vi "DIO64 Out Write.vi"(0 "board in":u16 format="%.0x", 5 "data":u16[][](array[numeric]) format="%.0x", 7 "Out Status":T1 {"startTime0" format="%.0x"; "startTime1" format="%.0x"; "cur trans" format="%.0x"; "cur reps" format="%.0x"; "#trans" format="%.0x"; "reps" format="%.0x"; "stopTime1" format="%.0x"; "stopTime0" format="%.0x"; "pktsize" format="%.0x"; "flags" format="%.0x"; "AICurrent" format="%.0x"; "startControl" format="%.0x"; "stopControl" format="%.0x"; "AIControl" format="%.0x"; "clkControl" format="%.0x"; "time0" format="%.0x"; "time1" format="%.0x"; "ticks" format="%.0x"; "readPtr" format="%.0x"; "writePtr" format="%.0x"; "fifo0" format="%.0x"; "fifoSize" format="%.0x"; "portCount" format="%.0x"}, 11 "error in (no error)":errorcluster) -> (4 "board out":u16 format="%.0x", 15 "error out":errorcluster)   [LabVIEW 2012]
doc: "DIO64 Out Write fills the output buffer with the data specified.\n\nCopyright (c) 2002 Viewpoint Systems Inc. All Rights Reserved"
uses:
  DIO64 Out Status.ctl
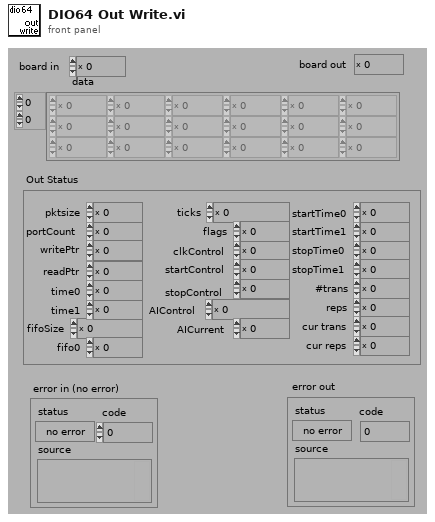
[diagram p1: front panel]
types:
  T1 = typedef "DIO64 Out Status.ctl" = cluster{"pktsize":u16, "portCount":u16, "writePtr":u16, "readPtr":u16, "time0":u16, "time1":u16, "fifoSize":u32, "fifo0":u16, "ticks":u32, "flags":u16, "clkControl":u16, "startControl":u16, "stopControl":u16, "AIControl":u32, "AICurrent":u16, "startTime0":u16, "startTime1":u16, "stopTime0":u16, "stopTime1":u16, "#trans":u16, "reps":u16, "cur trans":u16, "cur reps":u16}
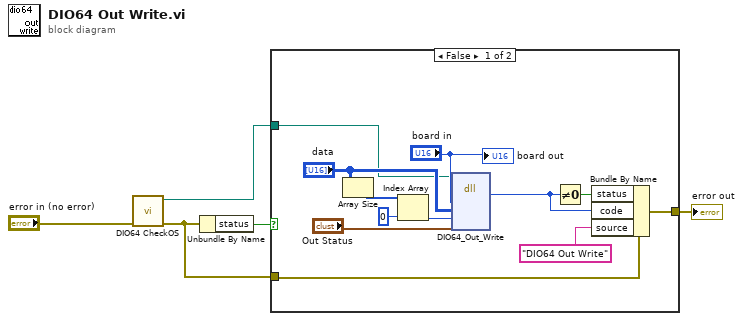
[diagram p0: block diagram]
diagram:
  n1 = call "DIO64 CheckOS.vi"("error in"="error in (no error)") -> ("error out"=w2:errorcluster, "path in"=w1:path)  [unwired: 9 in]
  n2 = Unbundle By Name(w2) -> ("status"=w5:bool)
  n3 = case shown="False" w5 {
    tunnel: w2 -> [w17 w18]
    tunnel: [w14 w18] -> w4
    tunnel: w1 -> [w6 _]
    frame False {
      n4 = Array Size(array="data") -> (size(s)=w9:i32[])
      n5 = Index Array(array=w9, index=0) -> (element=w10:i32)
      n6 = dll-call lib="C:/DIO64Visa/DLL/DIO64_Visa32/Debug/DIO64_Visa32.dll" fn="DIO64_Out_Write"(path in=w6, "board"="board in", "buffer"="data", "bufferSize"=w10, "status"="Out Status") -> ("return type"=w15:i32)  [unwired: 6 in, 2 out]
      n7 = Not Equal To 0?(x=w15) -> (x != 0?=w16:bool)
      n8 = Bundle By Name(cluster=w17, "status"=w16, "code"=w15, "source"="DIO64 Out Write") -> (w14:errorcluster)
      "board out" <- "board in"
    }
    frame True {
    }
  }
  "error out" <- w4
